vi "SolveIKPosition.vi"(0 "error in":errorcluster, 2 "Pose":T3={"Side"=enum."left", "Position"={"x"=0.457, "y"=-0.385, "z"=-0.261}, "Orientation (degrees)"={"Roll (y)"=3.13, "Pitch (x)"=-0.1, "Yaw (z)"=-1.85}}, 3 "node":string) -> (1 "error out":errorcluster, 4 "IK Reply":T1)   [LabVIEW 2015]
uses:
  ROS/Code/SubVIs/BaxterSide.ctl
  ROS/Code/Console/Servers/ServerSubs/TopicDef.ctl
  ROS/Code/SubVIs/_ROSDirection.ctl
  ROS/MessageBuilding/std_msgs/subs/u32Scalar.vi
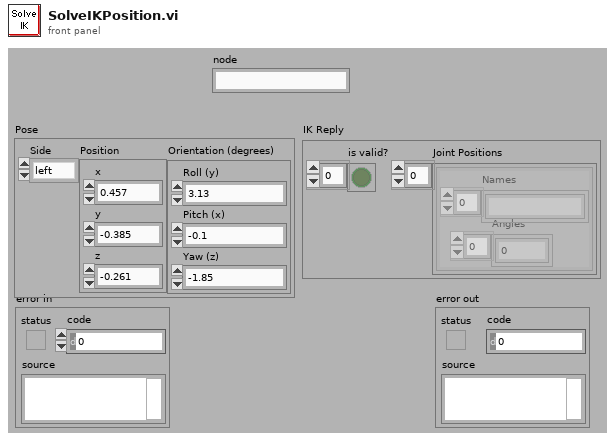
[diagram p1: front panel]
types:
  T1 = cluster{"is valid?":bool[], "Joint Positions":cluster{"Angles":dbl[], "Names":string[]}[]}
  T2 = typedef "BaxterSide.ctl" = enum16{"left", "right"}
  T3 = cluster{"Side":T2, "Position":cluster{"x":dbl, "y":dbl, "z":dbl}, "Orientation (degrees)":cluster{"Roll (y)":dbl, "Pitch (x)":dbl, "Yaw (z)":dbl}}
  T4 = typedef "TopicDef.ctl" = cluster{"Topic":string, "Type":string, "Action":T5, "Update (ms)":u16, "queue size":u16}
  T5 = typedef "_ROSDirection.ctl" = enum16{"Node", "Publisher", "Subscriber", "ServiceClient", "ServiceProvider"}
  T6 = cluster{"Roll (y)":dbl, "Pitch (x)":dbl, "Yaw (z)":dbl}
  T7 = typedef "_ROSControl.ctl" = cluster{"topic port":u16, "Node":string, "topic":string, "type":string, "node port":u16, "error ":errorcluster, "Direction":T5, "Update (ms)":u16, "FIFO size":u16}
  T8 = cluster{"Position":cluster{"x":dbl, "y":dbl, "z":dbl}, "Quaternion":cluster{"x":dbl, "y":dbl, "z":dbl, "w":dbl}}
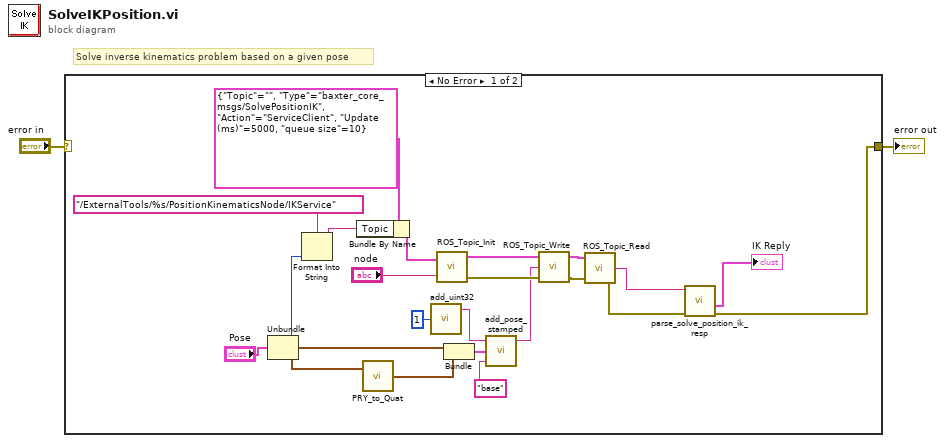
[diagram p0: block diagram]
diagram:
  # "Solve inverse kinematics problem based on a given pose"
  n1 = case shown="No Error" "error in" {
    selector: "error in" -> [_ w26]
    tunnel: [w6 w26] -> w2
    frame No Error {
      n2 = Unbundle("Pose") -> ("Side"=w5:T2, "Position"=w4:cluster{"x":dbl, "y":dbl, "z":dbl}, "Orientation (degrees)"=w3:T6)
      n3 = Format Into String(format string="/ExternalTools/%s/PositionKinematicsNode/IKService" ("topic"), w5) -> (resulting string=w14:string)  [unwired: 2 in, 1 out]
      n4 = Bundle By Name(cluster=T4 {"Topic"="", "Type"="baxter_core_msgs/SolvePositionIK", "Action"=enum."ServiceClient", "Update (ms)"=5000, "queue size"=10} ("Definitions"), "Topic"=w14) -> (w11:T4)
      n5 = call "PRY_to_Quat.vi"("Orientation"=w3) -> ("Quaternion"=w23:cluster{"x":dbl, "y":dbl, "z":dbl, "w":dbl})  [unwired: 1 in]
      n6 = call-poly "add_uint32.vi"("Numeric"=u32 1) -> ("msg out"=w19:string)  [unwired: 4 in]
      n7 = call "ROS_Topic_Init.vi"("Definitions"=w11, "node"="node") -> ("ROS out"=w18:T7, "error out"=w9:errorcluster)  [unwired: 1 in]
      n8 = Bundle("Position"=w4, "Quaternion"=w23) -> (w22:T8)  [unwired: 1 in]
      n9 = call "add_pose_stamped.vi"("frame_id"="base", "Pose"=w22, "msg in"=w19) -> ("msg out"=w8:string)  [unwired: 2 in]
      n10 = call "ROS_Topic_Write.vi"("error in (no error)"=w9, "Msg in"=w8, "ROS in"=w18) -> ("error out"=w10:errorcluster, "ROS out"=w15:T7)  [unwired: 1 in]
      n11 = call "ROS_Topic_Read.vi"("error in (no error)"=w10, "ROS in"=w15) -> ("error out"=w7:errorcluster, "Reply"=w17:string)  [unwired: 1 in, 1 out]
      n12 = call "parse_solve_position_ik_resp.vi"("error in"=w7, "msg in"=w17) -> ("error out"=w6:errorcluster, "IK Reply"=→"IK Reply":T1)  [unwired: 2 in, 2 out]
    }
    frame Error {
    }
  }
  "error out" <- w2
